vi "ASE Kalman Filter Simulation.vi"() -> ()   [LabVIEW 2018]
uses:
  <vilib>/Simulation/Scripting/Companion Diagram/SimConfigNode/SimParams.ctl
  <vilib>/Simulation/Scripting/Companion Diagram/SimConfigNode/_simSolvers.ctl
  <vilib>/Simulation/Implementation/Shared/SIMSCR Execution Mode.ctl
  <vilib>/Platform/TimedLoop/XDataNode/timing_clust.ctl
  <vilib>/Platform/TimedLoop/XDataNode/nitl_modes.ctl
  <vilib>/Platform/TimedLoop/XDataNode/wakeup.ctl
  <vilib>/Simulation/Param Hierarchy/Typedefs/SIMPH Param Control Actions.ctl
  <vilib>/addons/Control Design/_Stochastic Systems/Stochastic Systems.llb/Stochastic Systems SubVIs/cd_Second-Order Statistics Noise Model.ctl
  <vilib>/Simulation/Implementation/Shared/NILVSim_ParamChanged.vi
  <vilib>/Simulation/Implementation/Shared/NILVSim_FinishedLate.vi
  <vilib>/Simulation/Implementation/Shared/NILVSIM_BeginStep.vi
  <vilib>/Simulation/Utility/Implementation/SIM Halt.vi
  <vilib>/Simulation/DataSources/Implementation/NILVSim Signal Generator.llb/SIM Signal Generator (scalar).vi
  <vilib>/Simulation/Nonlinear/Implementation/NILVSim Saturation.llb/SIM Saturation (scalar).vi
  <vilib>/Simulation/ContinuousLinear/Implementation/NILVSim Transfer Function.llb/SIM Transfer Function Distributor (SISO).vi
  <vilib>/Simulation/ContinuousLinear/Implementation/NILVSim Transfer Function.llb/SIM Transfer Function Collector (SISO).vi
  <vilib>/Simulation/Nonlinear/Implementation/NILVSim RateLimiter.llb/SIM RateLimiter (scalar).vi
  <vilib>/Simulation/SignalDisplay/Implementation/NILVSim Time Waveform.llb/SIM Time Waveform (vector).vi
  <vilib>/Simulation/Utility/Implementation/NILVSim Memory.llb/NILVSim Memory (core).vi
  <vilib>/Simulation/ContinuousLinear/Implementation/NILVSim State Space.llb/SIM State Space Direct (CD).vi
  <vilib>/Simulation/SignalDisplay/Implementation/NILVSim Time Waveform.llb/SIM Time Waveform (scalar).vi
  <vilib>/Simulation/Implementation/Shared/NILVSim_Manager.vi
  <vilib>/Utility/error.llb/Clear Errors.vi
  <vilib>/Simulation/Implementation/Shared/NILVSim_FinalizeModel.vi
  <vilib>/imath/engines/lvmath2/RunTimeEngine/Managers/WorkSpace/UID Generator.vi
  <vilib>/imath/engines/lvmath2/RunTimeEngine/RunTimeType/NIMS_RunTimeType_From StrictType (excl LVString).vi
  <instcachedir>/0/NIMS_RunTimeType_From StrictType (excl LVString)_E7E34A65C99947108168652BAD14964D.lvgen/NIMS_RunTimeType_From StrictType (excl LVString)_E7E34A65C99947108168652BAD14964D_000.vi
  <vilib>/imath/engines/lvmath2/RunTimeEngine/LocalVariableDefStatement/MC_LocalVariableDefStatement_Display.vi
  <vilib>/imath/engines/lvmath/Plug In/Control Design/BuiltInFunctions/ss/NIMS_CD_ss(A,B,C,D).vi
  <vilib>/imath/engines/lvmath2/RunTimeEngine/Managers/SymbolTable/Clear UID.vi
  <vilib>/imath/engines/lvmath2/RunTimeEngine/NodeEndStatement/NIMS_NodeEndStatement_Output.vi
  <instcachedir>/0/NIMS_NodeEndStatement_Output_53EC0D466D134D7ABD903AC30B43404B.lvgen/NIMS_NodeEndStatement_Output_53EC0D466D134D7ABD903AC30B43404B_011.vi
  <instcachedir>/0/NIMS_NodeEndStatement_Output_53EC0D466D134D7ABD903AC30B43404B.lvgen/NIMS_NodeEndStatement_Output_53EC0D466D134D7ABD903AC30B43404B_010.vi
  <instcachedir>/0/NIMS_NodeEndStatement_Output_53EC0D466D134D7ABD903AC30B43404B.lvgen/NIMS_NodeEndStatement_Output_53EC0D466D134D7ABD903AC30B43404B_002.vi
  <vilib>/imath/engines/lvmath2/RunTimeEngine/ErrorHandling/NIMS_Finalize Error.vi
  <vilib>/addons/Control Design/_Utility/Model Viewer.llb/Model Viewer SubVI/cd_Draw State-Space Equation (SS).vi
  <vilib>/addons/Control Design/_Stochastic Systems/Stochastic Systems.llb/CD Construct Stochastic Model (Numeric).vi
  <vilib>/addons/Control Design/_Stochastic Systems/Stochastic Systems.llb/CD Construct Noise Model (Numeric).vi
  <vilib>/Simulation/Implementation/Shared/SIM Unbundle Sim Info.vi
  <vilib>/Simulation/Implementation/Shared/SIMSH Read Queue.vi
  <vilib>/Simulation/Implementation/Shared/NILVSim_Initialize.vi
  <vilib>/Simulation/Utility/Implementation/NILVSim Get Time and IsAcceptedStep.vi
  <vilib>/Simulation/Implementation/Shared/NILVSim_GetModelError.vi
  <vilib>/Simulation/Implementation/Shared/SIM Bundle Sim Info.vi
  <vilib>/Simulation/Scripting/Companion Diagram/SimConfigNode/SimDog.xnode
  <vilib>/addons/Control Design/_Model Construction/Model Typedefs.llb/CD State Space Model (MIMO).ctl
  <vilib>/addons/Control Design/_Model Construction/Model Typedefs.llb/CD General Elements.ctl
  <vilib>/addons/Control Design/_Implementation/CD Continuous Recursive Kalman Filter.vi
  <vilib>/Platform/TimedLoop/XDataNode/XDataNode.xnode
  <vilib>/Simulation/Implementation/XNodeFramework/SimXNode/SimX.xnode
  <vilib>/addons/Control Design/_Utility/NI_CD_Model Viewer.lvlib
  <vilib>/Simulation/ContinuousLinear/Implementation/NILVSim Transfer Function.llb/SIM Transfer Function (SISO).vi
  <vilib>/addons/Control Design/_Model Construction/NI_LinSys_Model Typedefs.lvlib
  <vilib>/addons/Control Design/_Stochastic Systems/NI_CD_Stochastic Systems.lvlib
  <vilib>/imath/engines/lvmath2/RunTimeEngine/Managers/SymbolTable/NIMS_WorkSpace.lvlib
  <vilib>/Platform/TimedLoop/XDataNode/XDNodeRunTimeDep.lvlib
  <vilib>/Simulation/Implementation/Shared/NI_SIM_Implementation.lvlib
panel:
  in  "R":dbl[][](array[numeric])=[[0.001, 0.0], [0.0, 0.001]] format="%#.5f"
  in  "Q":dbl[][](array[numeric])=[[0.001, 0.0, 0.0, 0.0], [0.0, 0.001, 0.0, 0.0], [0.0, 0.0, 0.001, 0.0], [0.0, 0.0, 0.0, 0.001]] format="%#.4f"
  out "Kalman Filter":waveform(dbl)[](graph)=[{"t0"=timestamp(9.964 s since 1904-01-01), "dt"=1.0, "Y"=[0.009999999999999988]}, {"t0"=timestamp(9.964 s since 1904-01-01), "dt"=1.0, "Y"=[0.0080681545382706]}, {"t0"=timestamp(9.964 s since 1904-01-01), "dt"=1.0, "Y"=[0.003319879208579203]}]
  out "Suspension Travel (m)":waveform(dbl)(graph)={"t0"=timestamp(9.964 s since 1904-01-01), "dt"=1.0, "Y"=[-0.004758345307169018]}
  in  "Setpoint Command":T1={"Amplitude (m)"=0.01, "Frequency (Hz)"=0.3} caption="Road (Bottom Plate)\nAmplitude Command (m)" {"Frequency (Hz)" min=0.0 max=0.5 step=0.009999999776482582 format="%_3f"; "Amplitude (m)" min=-10.0 max=10.0 step=0.5 format="%_3f"}
  out "Open Loop State-Space Model":picture
  out "Zr(m), Zs(m), Zus(m)":waveform(dbl)[](graph)=[{"t0"=timestamp(9.964 s since 1904-01-01), "dt"=1.0, "Y"=[0.009999999999999988]}, {"t0"=timestamp(9.964 s since 1904-01-01), "dt"=1.0, "Y"=[0.008101035650175014]}, {"t0"=timestamp(9.964 s since 1904-01-01), "dt"=1.0, "Y"=[0.0033426903430059957]}]
  out "Accelerometer Measurement (m/sec^2)":waveform(dbl)(graph)={"t0"=timestamp(9.964 s since 1904-01-01), "dt"=1.0, "Y"=[1.725866428659439]}
  in  "Stop Button":bool
  # "Active Suspension Kalman Filter Simulation"
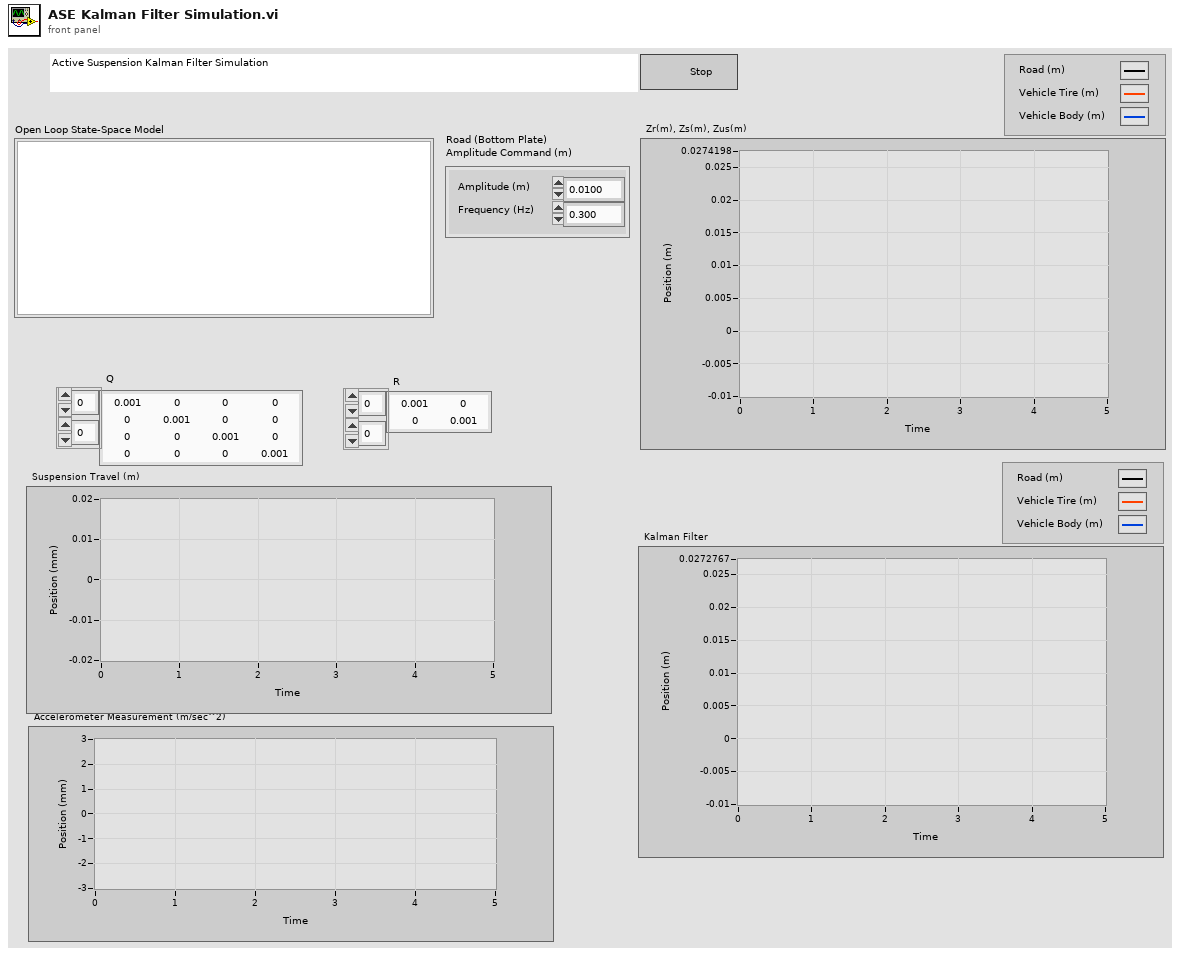
[diagram p1: front panel]
types:
  T1 = cluster{"Amplitude (m)":dbl, "Frequency (Hz)":dbl}
  T2 = typedef "NI_LinSys_Model Typedefs.lvlib/CD State Space Model (MIMO).ctl" = cluster{"properties":T3, "A":dbl[][], "B":dbl[][], "C":dbl[][], "D":dbl[][], "StateNames":string[], "Transport Delay":dbl[][]}
  T3 = typedef "NI_LinSys_Model Typedefs.lvlib/CD General Elements.ctl" = cluster{"Model name":string, "Input names":string[], "Output names":string[], "Input Delays":dbl[], "Output Delays":dbl[], "Sampling Time":dbl, "Notes":string}
  T4 = typedef "NI_CD_Stochastic Systems.lvlib/cd_Stochastic State-Space Model.ctl" = cluster{"Sampling Time (s)":dbl, "G":dbl[][], "B":dbl[][], "A":dbl[][], "C":dbl[][], "D":dbl[][], "H":dbl[][]}
  T5 = typedef "NI_CD_Stochastic Systems.lvlib/cd_Second-Order Statistics Noise Model.ctl" = cluster{"Q":dbl[][], "E{w}":dbl[], "E{v}":dbl[], "R":dbl[][], "N":dbl[][]}
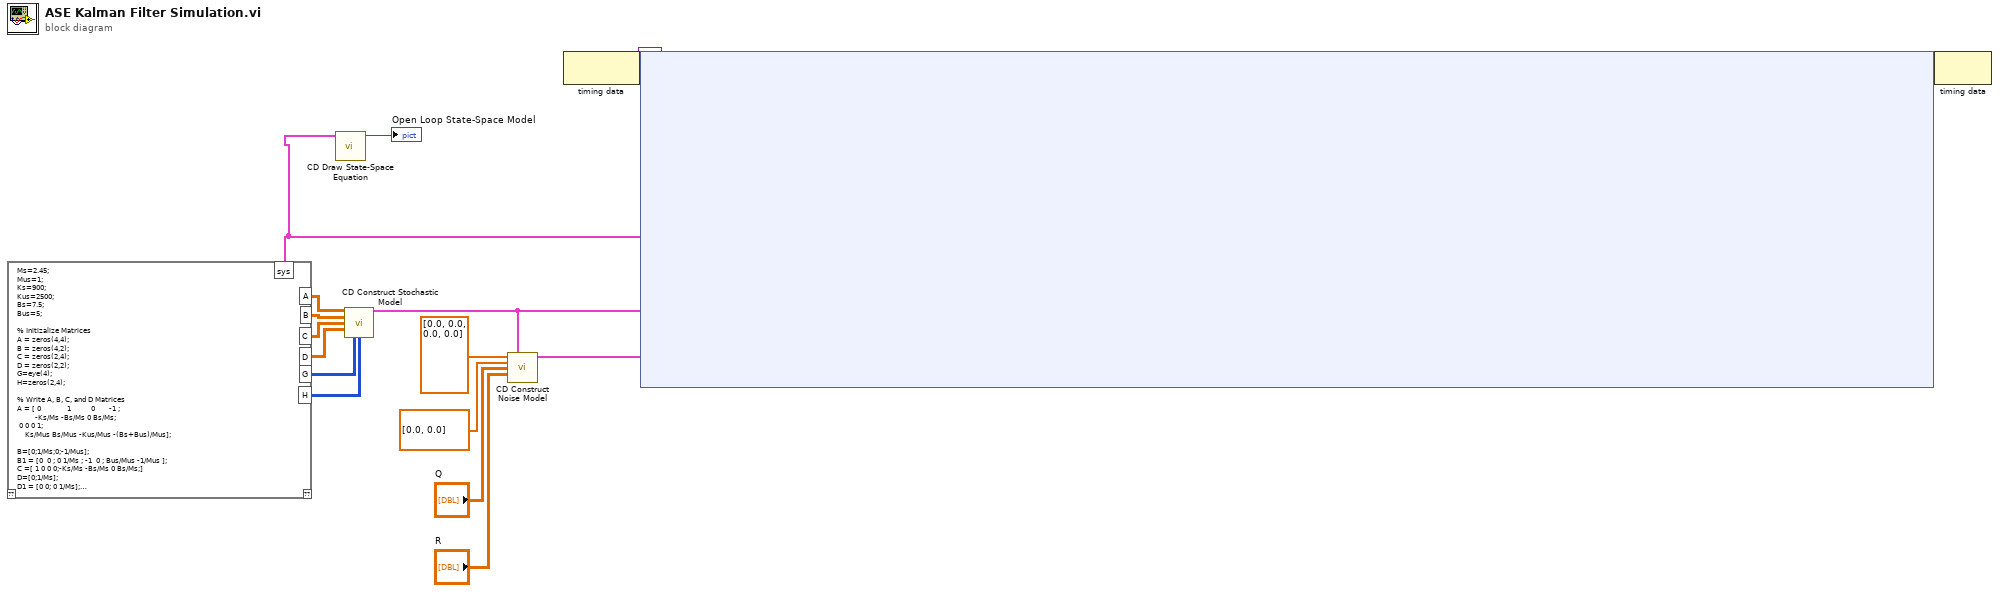
[diagram p0: block diagram]
diagram:
  n1 = mathscript code="Ms=2.45;\nMus=1;\nKs=900;\nKus=2500;\nBs=7.5;\nBus=5;\n\n% Initizalize Matrices\nA = zeros(4,4);\nB = zeros(4,2);\nC = zeros(2,4);\nD = zeros(2,2);\nG=eye(4);\nH=zeros(2,4);\n\n% Write A, B, C, and D Matrices\nA = [ 0             1          0       -1 ; \n         -Ks/Ms -Bs/Ms 0 Bs/Ms;  \n 0 0 0 1;\n    Ks/Mus Bs/Mus -Kus/Mus -(Bs+Bus)/Mus];\n\nB=[0;1/Ms;0;-1/Mus];\nB1 = [0  0 ; 0 1/Ms ; -1  0 ; Bus/Mus -1/Mus ];\nC =[ 1 0 0 0;-Ks/Ms -Bs/Ms 0 Bs/Ms;]\nD=[0;1/Ms];\nD1 = [0 0; 0 1/Ms];\n% Create State-Space Representation\nsys=ss(A,B1,C,D1);"() -> ("A"=w13:dbl[][], "B"=w11:dbl[][], "C"=w12:dbl[][], "D"=w10:dbl[][], "G"=w7:i32[][], "H"=w6:i32[][], "sys"=w1:T2)  [unwired: 1 in, 1 out]
  n2 = call-poly <vilib>:"CD Draw State-Space Equation.vi"("State-Space Model"=w1) -> ("Equation"=→"Open Loop State-Space Model":picture)  [unwired: 8 in, 2 out]
  n3 = call-poly <vilib>:"CD Construct Stochastic Model.vi"("A"=w13, "B"=w11, "C"=w12, "D"=w10, "G"=w7, "H"=w6) -> ("Stochastic State-Space Model"=w2:T4)  [unwired: 2 in, 7 out]
  n4 = call-poly <vilib>:"CD Construct Noise Model.vi"("E{w}"=dbl[] [0.0, 0.0, 0.0, 0.0], "Stochastic State-Space Model"=w2, "E{v}"=dbl[] [0.0, 0.0], "Q"="Q", "R"="R") -> ("Second-Order Statistics Noise Model out"=w5:T5)  [unwired: 9 in, 1 out]
  n5 = node-c288() -> (w16:variant)  [unwired: 1 in]
  n6 = node-c254 ("Control & Simulation Loop")(w16, w1, w2, w5) -> (w15:variant)
  n7 = node-c288(w15) -> ()  [unwired: 1 out]
